vi "error cluster from custom error code.vi"(5 "is warning? (True)":bool=TRUE, 6 "string values":string[](array[string]), 7 "show call chain? (True)":bool=TRUE, 8 "error in":errorcluster, 9 "keys":string[](array[string]), 10 "error message":string="The specified target is unsupported. SMI is only intended for real-time targets.", 11 "custom error code (0)":i32) -> (0 "error out":errorcluster)   [LabVIEW 2014, in "SMI.lvlib"]
uses:
  SMI.lvlib
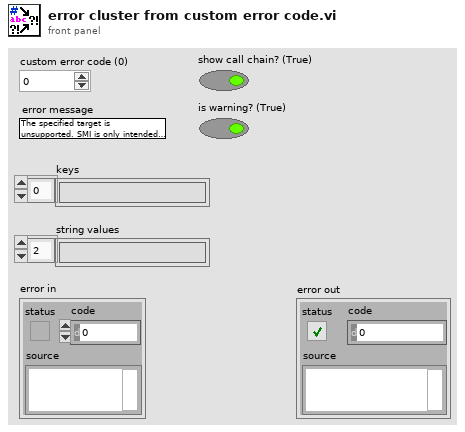
[diagram p1: front panel]
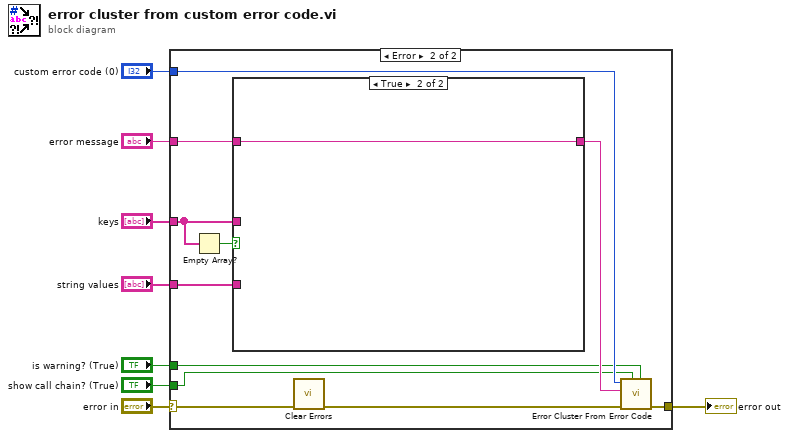
[diagram p0: block diagram]
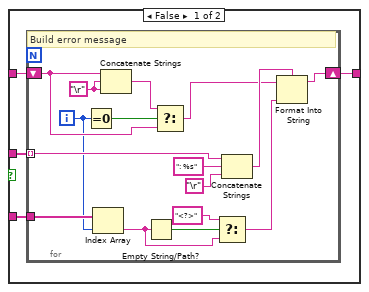
[diagram p3: hidden frame]
diagram:
  n1 = case shown="Error" "error in" {
    selector: "error in" -> [w9 w16]
    tunnel: "error message" -> [_ w20]
    tunnel: "keys" -> [_ w11]
    tunnel: "string values" -> [_ w19]
    tunnel: "custom error code (0)" -> [_ w17]
    tunnel: "is warning? (True)" -> [_ w14]
    tunnel: "show call chain? (True)" -> [_ w13]
    tunnel: [w9 w12] -> w1
    frame No Error {
    }
    frame Error {
      n2 = Empty Array?(array=w11) -> (empty?=w10:bool)
      n3 = case shown="True" w10 {
        tunnel: w20 -> [w24 w41]
        tunnel: w19 -> [w23 _]
        tunnel: [w22 w41] -> w18
        tunnel: w11 -> [w21 _]
        frame False {
          n4 = for {
            shift-right: [w40] -> w22
            shift-left: w24 -> [w33]
            tunnel: w21 -> [w37] mode=indexing
            tunnel: w23 -> [w30]
            i -> [w29]
            w35 = "\r"
            # "Build error message"
            n5 = Equal To 0?(x=w29) -> (x = 0?=w34:bool)
            n6 = Index Array(array=w30, index=w29) -> (element=w26:string)
            n7 = Concatenate Strings(w33, w35, w35) -> (w32:string)
            n8 = Empty String/Path?(string/path=w26) -> (empty?=w28:bool)
            n9 = Select(t=w32, s=w34, f=w33) -> (s? t:f=w31:string)
            n10 = Select(t="<?>", s=w28, f=w26) -> (s? t:f=w25:string)
            n11 = Concatenate Strings(w37, ": %s", "\r") -> (w36:string)
            n12 = Format Into String(format string=w36, initial string=w31, w25) -> (resulting string=w40:string)  [unwired: 1 in, 1 out]
          }
        }
        frame True {
        }
      }
      n13 = call <vilib>:"Clear Errors.vi"("error in (no error)"=w16) -> ("error out"=w15:errorcluster)  [unwired: 5 in, 1 out]
      n14 = call <vilib>:"Error Cluster From Error Code.vi"("is warning? (False)"=w14, "show call chain? (False)"=w13, "error in (no error)"=w15, "error message (\"\")"=w18, "error code (0)"=w17) -> ("error out"=w12:errorcluster)  [unwired: 4 in]
    }
  }
  "error out" <- w1
